vi "forwardByNavX_theSide(queuesWithNavX).vi"(8 "error in (no error)":errorcluster, 11 "distance the side":u32) -> (0 "error out":errorcluster)   [LabVIEW 2017]
uses:
  <vilib>/myRIO/Instrument Drivers/Onboard IO/I2C/typedefs/I2C Reference.ctl
  <vilib>/myRIO/Common/Instrument Driver Framework/Utilities/typedefs/myRIO Generic Hardware Reference.ctl
  <vilib>/myRIO/Common/Instrument Driver Framework/Utilities/typedefs/Hardware Version Enum.ctl
  <vilib>/myRIO/Common/Instrument Driver Framework/Utilities/typedefs/myRIO v1.0 Reference.ctl
  <vilib>/myRIO/Common/Instrument Driver Framework/Utilities/typedefs/Generic FPGA Reference.ctl
  <vilib>/myRIO/Common/Instrument Driver Framework/myRIO v1.0/I2C/typedefs/I2C Channels Enum.ctl
  <vilib>/myRIO/Instrument Drivers/Onboard IO/I2C/typedefs/I2C Configuration.ctl
  <vilib>/myRIO/Instrument Drivers/Onboard IO/I2C/typedefs/I2C Transfer Rate.ctl
  <vilib>/userdefined/High Color/nirio_resource_hc.ctl
  <vilib>/myRIO/Common/Instrument Driver Framework/myRIO v1.0/I2C/vis/myRIO v1.1 Open I2C.vi
  <vilib>/myRIO/Common/Instrument Driver Framework/Utilities/vis/Validate Channels.vi
  <vilib>/myRIO/Common/Instrument Driver Framework/myRIO v1.0/I2C/vis/myRIO v1.0 Reserve I2C.vi
  <vilib>/myRIO/Common/Instrument Driver Framework/myRIO v1.0/I2C/vis/myRIO v1.0 Close I2C.vi
  <vilib>/myRIO/Common/Instrument Driver Framework/myRIO v1.0/I2C/vis/myRIO v1.0 Build MUX Configuration I2C.vi
  <vilib>/myRIO/Common/Instrument Driver Framework/myRIO v1.0/Resource Manager/vis/myRIO v1.0 Reserve Channel List.vi
  <vilib>/myRIO/Common/Instrument Driver Framework/myRIO v1.0/I2C/vis/myRIO v1.0 Unreserve I2C.vi
  <vilib>/myRIO/Common/Instrument Driver Framework/myRIO v1.0/Resource Manager/vis/myRIO v1.0 Create Configuration List.vi
  <vilib>/myRIO/Common/Instrument Driver Framework/myRIO v1.0/Resource Manager/vis/myRIO v1.0 Reserve Channel.vi
  <vilib>/myRIO/Common/Instrument Driver Framework/myRIO v1.0/Resource Manager/vis/myRIO v1.0 Unreserve Channel.vi
  <vilib>/myRIO/Common/Instrument Driver Framework/myRIO v1.0/Resource Manager/vis/myRIO v1.0 Unreserve Channel List.vi
  <vilib>/myRIO/Common/Instrument Driver Framework/myRIO v1.0/Resource Manager/vis/myRIO v1.0 Build Mutex Name.vi
  <vilib>/Utility/VariantDataType/GetNumericInfo.vi
  <vilib>/Utility/error.llb/Error Cluster From Error Code.vi
  <vilib>/myRIO/Common/Instrument Driver Framework/myRIO v1.0/myRIO v1.1 Open.vi
  <vilib>/myRIO/Common/Instrument Driver Framework/Utilities/vis/IO Manager.vi
  <vilib>/myRIO/Common/Instrument Driver Framework/Utilities/vis/Configuration Manager.vi
  <vilib>/myRIO/Common/Instrument Driver Framework/myRIO v1.0/Resource Manager/vis/myRIO v1.0 Configure IO.vi
  <vilib>/myRIO/Common/Instrument Driver Framework/myRIO v1.0/myRIO v1.0 Close.vi
  <vilib>/Instr/_visa.llb/VISA Configure Serial Port (Instr).vi
  <vilib>/myRIO/Common/Instrument Driver Framework/myRIO v1.0/DIO/vis/myRIO v1.0 Write DIO.vi
  <vilib>/myRIO/Common/Instrument Driver Framework/myRIO v1.0/I2C/vis/myRIO v1.0 Shutdown I2C.vi
  <vilib>/myRIO/Instrument Drivers/Onboard IO/I2C/vis/myRIO I2C Open.xnode
  <vilib>/myRIO/Instrument Drivers/Onboard IO/I2C/I2C.lvlib
  <vilib>/myRIO/Instrument Drivers/Onboard IO/DIO/DIO.lvlib
panel:
  out "output 1":u32
  out "axis Z(paste)":ext
  out "main angle":ext
  out "right":dbl
  out "left":dbl
  out "zero angle":ext
  in  "Stop Button":bool
  out "axis Z(after)":ext
  # "--- отклонения от нулевого угла"
  # "PWM"
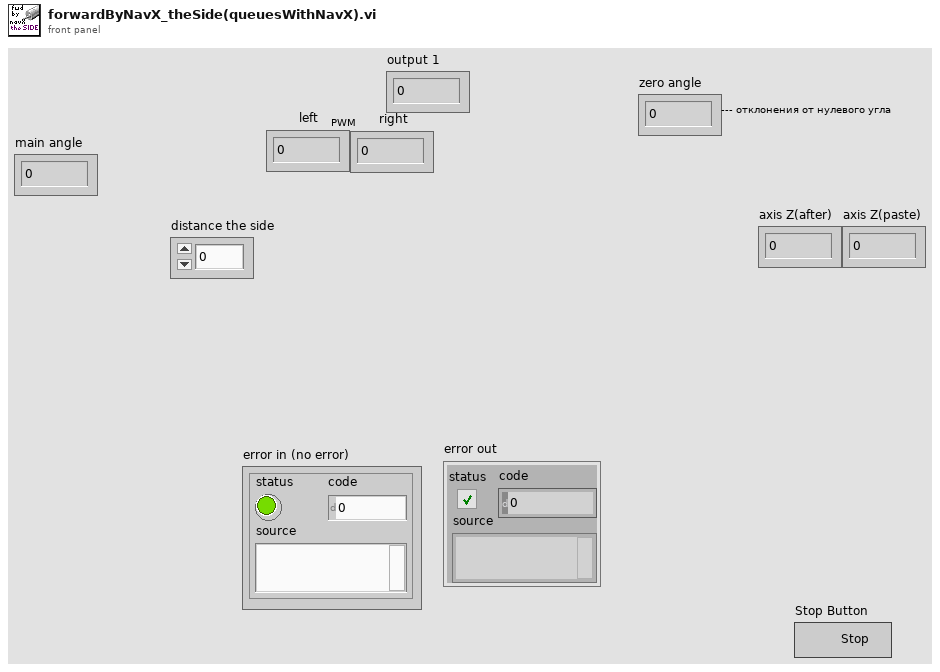
[diagram p1: front panel]
types:
  T1 = typedef "DIO.lvlib/DIO Reference.ctl" = cluster{"myRIO Reference":T2, "DIO Channels List":T6}
  T2 = typedef "myRIO Generic Hardware Reference.ctl" = cluster{"myRIO Model":T3, "myRIO Hardware Reference":T4}
  T3 = typedef "Hardware Version Enum.ctl" = enum16{"Unknown", "myRIO-1900", "myRIO-1950", "roboRIO", "NI ELVIS RIO CM"}
  T4 = typedef "myRIO v1.0 Reference.ctl" = cluster{"Generic FPGA Reference":T5, "Allow multiple opens":bool}
  T5 = typedef "Generic FPGA Reference.ctl" = refnum<k20>
  T6 = typedef "DIO Channels List.ctl" = T7[]
  T7 = typedef "DIO Channels Enum.ctl" = enum16{"Not Connected", "C/DIO0", "C/DIO1", "C/DIO2", "C/DIO3", "C/DIO4", "C/DIO5", "C/DIO6", "C/DIO7", "A/DIO0", "A/DIO1", "A/DIO2", "A/DIO3", "A/DIO4", "A/DIO5", "A/DIO6", "A/DIO7", "A/DIO8", "A/DIO9", "A/DIO10", "A/DIO11", "A/DIO12", "A/DIO13", "A/DIO14", "A/DIO15", "B/DIO0", "B/DIO1", "B/DIO2", "B/DIO3", "B/DIO4", "B/DIO5", "B/DIO6", "B/DIO7", "B/DIO8", "B/DIO9", "B/DIO10", "B/DIO11", "B/DIO12", "B/DIO13", "B/DIO14", "B/DIO15", "LED0", "LED1", "LED2", "LED3", "Button0", "DIO/DIO0", "DIO/DIO1", "DIO/DIO2", "DIO/DIO3", "DIO/DIO4", "DIO/DIO5", "DIO/DIO6", "DIO/DIO7", "DIO/DIO8", "DIO/DIO9", "SPI/CS0", "SPI/CS1", "SPI/CS2", "SPI/CS3", "LED RADIO (Green)", "LED RADIO (Red)", "LED COMM (Green)", "LED COMM (Red)", "LED MODE (Green)", "LED MODE (Red)"}
  T8 = typedef "I2C.lvlib/I2C Reference.ctl" = cluster{"myRIO Reference":T2, "I2C Channels Enum":T9, "I2C Configuration":T10}
  T9 = typedef "I2C Channels Enum.ctl" = enum16{"Not Connected", "A/I2C", "B/I2C", "I2C/I2C"}
  T10 = typedef "I2C.lvlib/I2C Configuration.ctl" = cluster{"I2C Transfer Rate":T11}
  T11 = typedef "I2C.lvlib/I2C Transfer Rate.ctl" = enum16{"Standard mode (100 kbps)", "Fast mode (400 kbps)"}
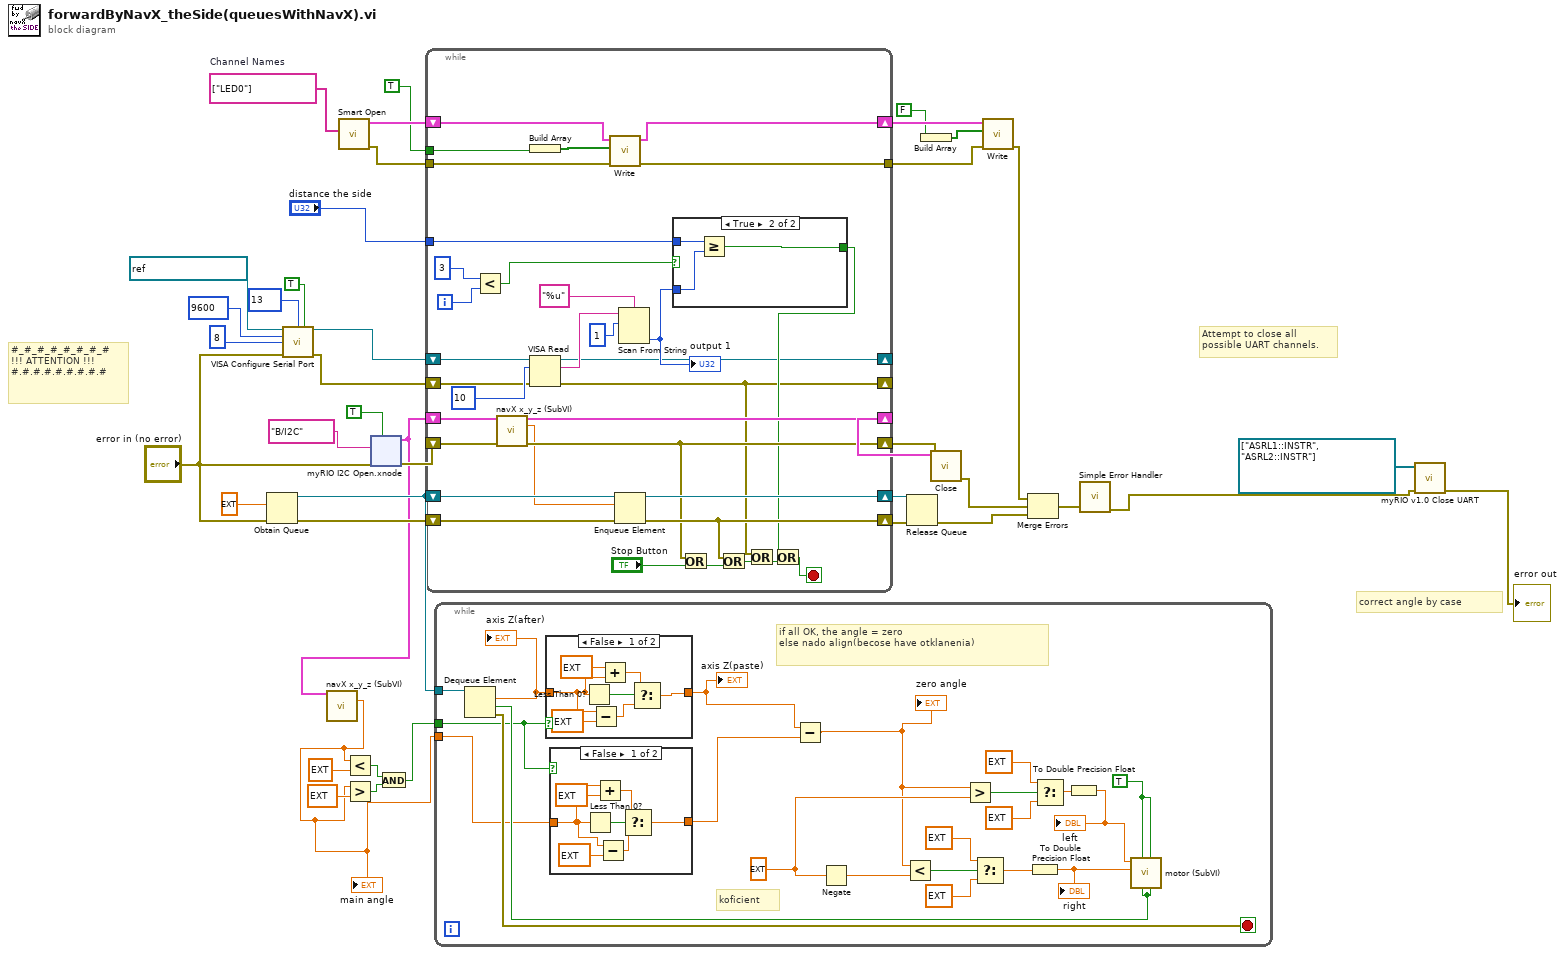
[diagram p0: block diagram]
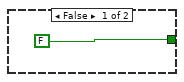
[diagram p4: hidden frame]
diagram:
  w9 = tag[] ["LED0"]  # Channel Names
  # "Attempt to close all possible UART channels."
  # "correct angle by case"
  # "#_#_#_#_#_#_#_#\n!!! ATTENTION !!!\n#.#.#.#.#.#.#.#.#"
  n1 = Obtain Queue(element data type=ext 0.0 ("value Z"), error in (no error)="error in (no error)") -> (queue out=w29:refnum<queue>, error out=w41:errorcluster)  [unwired: 3 in, 1 out]
  n2 = call-poly "VISA Configure Serial Port"("VISA resource name"=refnum<visa-resource-name> "ASRL2::INSTR" ("UART selector"), "termination char\n(0xA = '\\n' = LF)"=u8 13 ("termination char = CR"), "Enable Termination\nChar (T)"=TRUE ("enable termination char"), "baud rate (9600)"=u32 9600 ("baud rate"), "data bits (8)"=u16 8 ("data bits"), "error in (no error)"="error in (no error)") -> ("VISA resource name out"=w15:refnum<visa-resource-name>, "error out"=w16:errorcluster)  [unwired: 8 in]
  n3 = call <vilib>:"Smart Open.vi"("Channel Names"=w9) -> ("error out"=w7:errorcluster, "DIO Ref Out"=w8:T1)  [unwired: 9 in]
  n4 = xnode "myRIO I2C Open.xnode"("error in (no error)"="error in (no error)", "Allow multiple opens?"=TRUE, "Channel Name"=tag "B/I2C") -> ("error out"=w34:errorcluster, "I2C Ref Out"=w28:T8)
  n5 = call "navX x_y_z (SubVI).vi"("I2C Ref Out in"=w28) -> ("value Z"=w25:ext)  [unwired: 10 in, 4 out]
  "main angle" <- w25
  n6 = Less?(x=w25, y=ext 90.0) -> (x < y?=w23:bool)
  n7 = Greater?(x=w25, y=ext -90.0) -> (0:w26:bool)
  n8 = And(x=w23, y=w26) -> (x .and. y?=w22:bool)
  n9 = while {
    shift-right: [w69] -> w39
    shift-left: w41 -> [w74]
    shift-right: [w73] -> w40
    shift-left: w29 -> [w75]
    shift-right: [w70] -> w35
    shift-left: w28 -> [w71]
    shift-right: [w66] -> w33
    shift-left: w34 -> [w67]
    tunnel: "distance the side" -> [w53]
    shift-right: [w49] -> _
    shift-left: w16 -> [w55]
    shift-right: [w51] -> _
    shift-left: w15 -> [w54]
    tunnel: w7 -> [w45]
    tunnel: TRUE -> [w44]
    tunnel: [w42] -> w2
    shift-right: [w43] -> w5
    shift-left: w8 -> [w46]
    i -> [w48]
    stop <- w63 stop-if-true
    n10 = Less?(x=3, y=w48) -> (x < y?=w56:bool)
    n11 = call "navX x_y_z (SubVI).vi"("I2C Ref Out in"=w71, "error in (no error)"=w67) -> ("I2C Ref Out out"=w70:T8, "value Z"=w65:ext, "error out"=w66:errorcluster)  [unwired: 9 in, 2 out]
    n12 = Build Array(w44) -> (w47:bool[])
    n13 = VISA Read(VISA resource name=w54, byte count=u32 10, error in (no error)=w55) -> (VISA resource name out=w51:refnum<visa-resource-name>, read buffer=w59:string, error out=w49:errorcluster)  [unwired: 1 out]
    n14 = call <vilib>:"Write.vi"("error in (no error)"=w45, "Values"=w47, "DIO Ref In"=w46) -> ("error out"=w42:errorcluster, "DIO Ref Out"=w43:T1)  [unwired: 6 in]
    n15 = Enqueue Element(queue=w75, element=w65, error in (no error)=w74) -> (queue out=w73:refnum<queue>, error out=w69:errorcluster)  [unwired: 1 in, 1 out]
    n16 = Scan From String(format string="%u", input string=w59, initial scan location=u32 1) -> (output 1=w58:u32)  [unwired: 2 in, 3 out]
    "output 1" <- w58
    n17 = case shown="True" w56 {
      tunnel: w58 -> [_ w79]
      tunnel: w53 -> [_ w78]
      tunnel: [FALSE w77] -> w52
      frame False {
      }
      frame True {
        n18 = Greater Or Equal?(x=w78, y=w79) -> (x >= y?=w77:bool)
      }
    }
    n19 = Or(x=w66, y="Stop Button") -> (x .or. y?=w68:bool)
    n20 = Or(x=w69, y=w68) -> (x .or. y?=w64:bool)
    n21 = Or(x=w49, y=w64) -> (x .or. y?=w50:bool)
    n22 = Or(x=w52, y=w50) -> (x .or. y?=w63:bool)
  }
  n23 = while {
    tunnel: w29 -> [w101]
    tunnel: w25 -> [w83]
    tunnel: w22 -> [w82]
    stop <- w100 stop-if-true
    w89 = TRUE ("M0 (Pin 21)")
    w93 = ext 1.0 ("y")
    # "koficient"
    # "if all OK, the angle = zero\nelse nado align(becose have otklanenia)"
    n24 = Dequeue Element(queue=w101) -> (element=w85:ext, timed out?=w88:bool, error out=w100:errorcluster)  [unwired: 2 in, 1 out]
    "axis Z(after)" <- w85
    n25 = case shown="False" w82 {
      tunnel: [w115 w117] -> w86
      tunnel: w85 -> [w111 w117]
      frame False {
        n26 = Less Than 0?(x=w111) -> (x < 0?=w116:bool)
        n27 = Subtract(x=w111, y=ext 180.0) -> (x-y=w112:ext)
        n28 = Add(x=ext 180.0, y=w111) -> (x+y=w114:ext)
        n29 = Select(t=w114, s=w116, f=w112) -> (s? t:f=w115:ext)
      }
      frame True {
      }
    }
    "axis Z(paste)" <- w86
    n30 = case shown="False" w82 {
      tunnel: [w107 w109] -> w84
      tunnel: w83 -> [w104 w109]
      frame False {
        n31 = Less Than 0?(x=w104) -> (x < 0?=w108:bool)
        n32 = Add(x=w104, y=ext 180.0) -> (x+y=w106:ext)
        n33 = Subtract(x=w104, y=ext 180.0) -> (x-y=w105:ext)
        n34 = Select(t=w106, s=w108, f=w105) -> (s? t:f=w107:ext)
      }
      frame True {
      }
    }
    n35 = Subtract(x=w86, y=w84) -> (x-y=w87:ext)
    "zero angle" <- w87
    n36 = Negate(x=w93) -> (-x=w92:ext)
    n37 = Less?(x=w87, y=w92) -> (x < y?=w96:bool)
    n38 = Greater?(x=w87, y=w93) -> (0:w99:bool)
    n39 = Select(t=ext 0.2 ("y"), s=w96, f=ext 0.4 ("y")) -> (s? t:f=w90:ext)
    n40 = To Double Precision Float(number=w90) -> (double precision float=w81:dbl)
    "right" <- w81
    n41 = Select(t=ext 0.2 ("y"), s=w99, f=ext 0.4 ("y")) -> (s? t:f=w91:ext)
    n42 = To Double Precision Float(number=w91) -> (double precision float=w80:dbl)
    "left" <- w80
    n43 = call "motor (SubVI).vi"("M1 (Pin 26)"=w88, "M1 (Pin 25)"=w89, "M0 (Pin 23)"=w88, "M0 (Pin 21)"=w89, "PWM1"=w81, "PWM0"=w80) -> ()  [unwired: 5 in, 1 out]
  }
  n44 = Release Queue(queue=w40, error in (no error)=w39) -> (error out=w30:errorcluster)  [unwired: 1 in, 2 out]
  n45 = Build Array(FALSE) -> (w4:bool[])
  n46 = call <vilib>:"Close.vi"("error in (no error)"=w33, "I2C Ref In"=w35) -> ("error out"=w31:errorcluster)  [unwired: 9 in]
  n47 = call <vilib>:"Write.vi"("error in (no error)"=w2, "Values"=w4, "DIO Ref In"=w5) -> ("error out"=w1:errorcluster)  [unwired: 6 in, 1 out]
  n48 = Merge Errors(w1, w31, w30) -> (w32:errorcluster)
  n49 = call <vilib>:"Simple Error Handler.vi"("error in (no error)"=w32) -> ("error out"=w12:errorcluster)  [unwired: 4 in, 4 out]
  n50 = call <vilib>:"myRIO v1.0 Close UART.vi"("error in (no error)"=w12, "VISA resource array"=refnum<visa-resource-name>[] ["ASRL1::INSTR", "ASRL2::INSTR"]) -> ("error out"=→"error out":errorcluster)  [unwired: 9 in]
